vi "direction_channel_consumer.vi"(6 "Sampling Frequency [Hz]":dbl, 8 "error in (no error)":errorcluster, 10 "Sampling Offset [s]":dbl, 11 "Q":refnum<queue>) -> (0 "error out":errorcluster, 3 "Direction":i64)   [LabVIEW 2025, in "LabJackEKG.lvlib"]
uses:
  LabJackEKG.lvlib
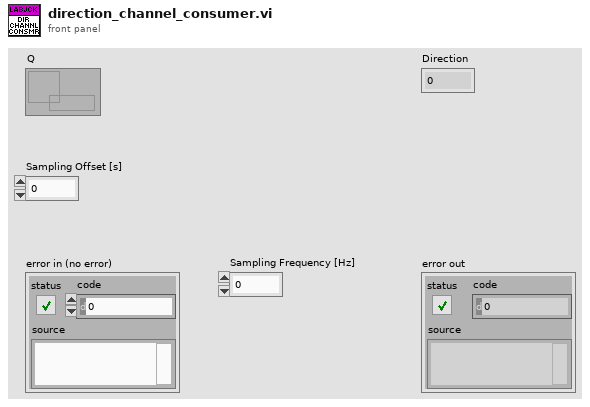
[diagram p1: front panel]
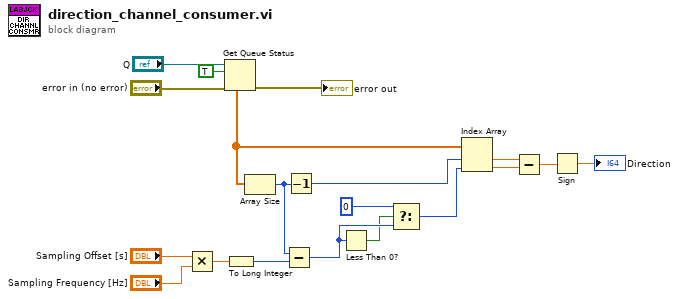
[diagram p0: block diagram]
diagram:
  n1 = Multiply(x="Sampling Offset [s]", y="Sampling Frequency [Hz]") -> (x*y=w17:dbl)
  n2 = Get Queue Status(queue="Q", return elements? (F)=TRUE, error in (no error)="error in (no error)") -> (error out=→"error out":errorcluster, elements=w11:dbl[])  [unwired: 6 out]
  n3 = To Long Integer(number=w17) -> (32bit integer=w10:i32)
  n4 = Array Size(array=w11) -> (size(s)=w9:i32)
  n5 = Subtract(x=w9, y=w10) -> (x-y=w6:i32)
  n6 = Decrement(x=w9) -> (x-1=w19:i32)
  n7 = Less Than 0?(x=w6) -> (x < 0?=w5:bool)
  n8 = Select(t=0, s=w5, f=w6) -> (s? t:f=w7:i32)
  n9 = Index Array(array=w11, index #1=w19, index #2=w7) -> (element #1=w13:dbl, element #2=w8:dbl)
  n10 = Subtract(x=w13, y=w8) -> (x-y=w3:dbl)
  n11 = Sign(1:w3) -> (0:→"Direction":dbl)
